vi "ServerUDP_Arduino-Labview.vi"() -> ()   [LabVIEW 2014]
doc: "The UDP protocol differs from TCP in that there is no error-checking with the packets of information that are sent, and thus no guarantee whatsoever that an intended recipient will actually receive a given piece of data.\n\nUDP does offer the ability to \"broadcast\" data across a network--simply specify an IP Address of all ones (255.255.255.255) to attempt to broadcast information network-wide. Keep in mind that routers and other network hardware will generally refuse to forward the broadcast beyond certain points, so the extent of the broadcast will in practice be limited."
panel:
  in  "stop":bool
  out "y":dbl
  out "x":dbl
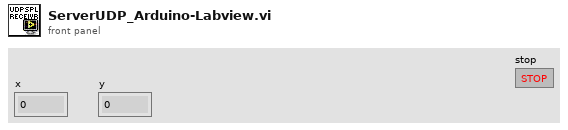
[diagram p1: front panel]
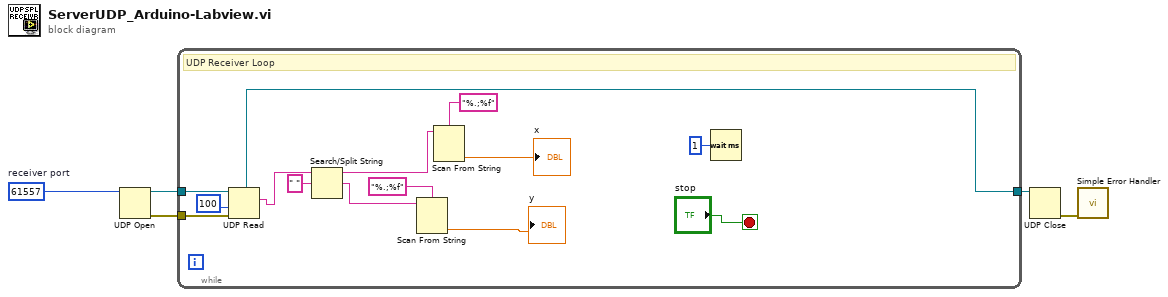
[diagram p0: block diagram]
diagram:
  w1 = u16 61557  # receiver port
  n1 = UDP Open(11:w1) -> (port=w2:refnum<k16>, 0:w3:errorcluster)  [unwired: 4 in, 1 out]
  n2 = while {
    tunnel: w2 -> [w19]
    tunnel: [w16] -> w5
    tunnel: w3 -> [w18]
    stop <- "stop" stop-if-true
    # "UDP Receiver Loop"
    n3 = UDP Read(connection ID=w19, timeout ms (25000)=100, 8:w18) -> (data out=w10:string, 3:w16:refnum<k16>)  [unwired: 4 out]
    n4 = Search/Split String(string=w10, search string/char (-)=" ") -> (substring before match=w12:string, match + rest of string=w11:string)  [unwired: 1 in, 1 out]
    n5 = Scan From String(format string="%.;%f", input string=w11) -> (output 1=→"y":dbl)  [unwired: 3 in, 3 out]
    n6 = Scan From String(format string="%.;%f", input string=w12) -> (output 1=→"x":dbl)  [unwired: 3 in, 3 out]
    n7 = Wait (ms)(milliseconds to wait=u32 1) -> ()  [unwired: 1 out]
  }
  n8 = UDP Close(connection ID=w5) -> (error out=w4:errorcluster)  [unwired: 1 in, 1 out]
  n9 = call <vilib>:"Simple Error Handler.vi"("error in (no error)"=w4) -> ()  [unwired: 1 in, 8 out]
